vi "Update Digital Audio Generation (Freq and Amp)(N Chan).vi"(8 "error in (no error)":errorcluster, 9 "gain":dbl[](array[numeric]), 10 "frequency":dbl[](array[numeric]), 11 "PCM tasks":T1) -> (0 "error out":errorcluster, 3 "PCM tasks":T1)   [LabVIEW 2021]
uses:
  controls/digital audio protocol/PCM tasks.ctl
  <vilib>/PDM Acquisition Toolkit/host/Classes/Tasks/PCM Output/Controls/PCM Output Task DVR.ctl
  <vilib>/PDM Acquisition Toolkit/host/Classes/Tasks/PCM Output/PCM Output Task.lvclass
  C:/Program Files/National Instruments/LabVIEW 2021/vi.lib/PDM Acquisition Toolkit/host/Classes/Tasks/Parent/DecoderTask.lvclass
  <vilib>/PDM Acquisition Toolkit/host/Classes/Channels/PCM Output/PCM Output Channel.lvclass
  C:/Program Files/National Instruments/LabVIEW 2021/vi.lib/PDM Acquisition Toolkit/host/Classes/Channels/DecoderChannel.lvclass
  <vilib>/PDM Acquisition Toolkit/host/Classes/Channels/PCM Output/controls/PCM Output Channel - Signal Properties.ctl
  <vilib>/PDM Acquisition Toolkit/host/Classes/Channels/DecoderChannel.lvclass
  C:/Program Files/National Instruments/LabVIEW 2021/vi.lib/PDM Acquisition Toolkit/host/Classes/Channels/PCM Output/PCM Output Channel.lvclass
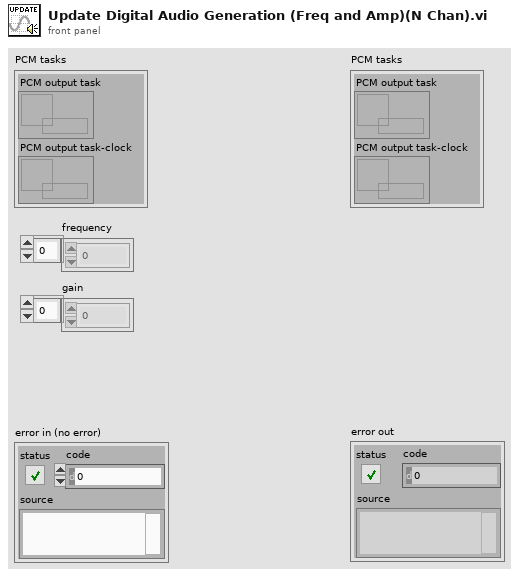
[diagram p1: front panel]
types:
  T1 = typedef "PCM tasks.ctl" = cluster{"PCM output task":T2, "PCM output task-clock":T2}
  T2 = typedef "PDM Acquisition Class Library.lvlib/PCM Output Task.lvclass/PCM Output Task DVR.ctl" = refnum<data-value>
  T3 = typedef "PDM Acquisition Class Library.lvlib/PCM Output Channel.lvclass/PCM Output Channel - Signal Properties.ctl" = cluster{"cyclic period":dbl, "cyclic phase offset":dbl, "gain":dbl}
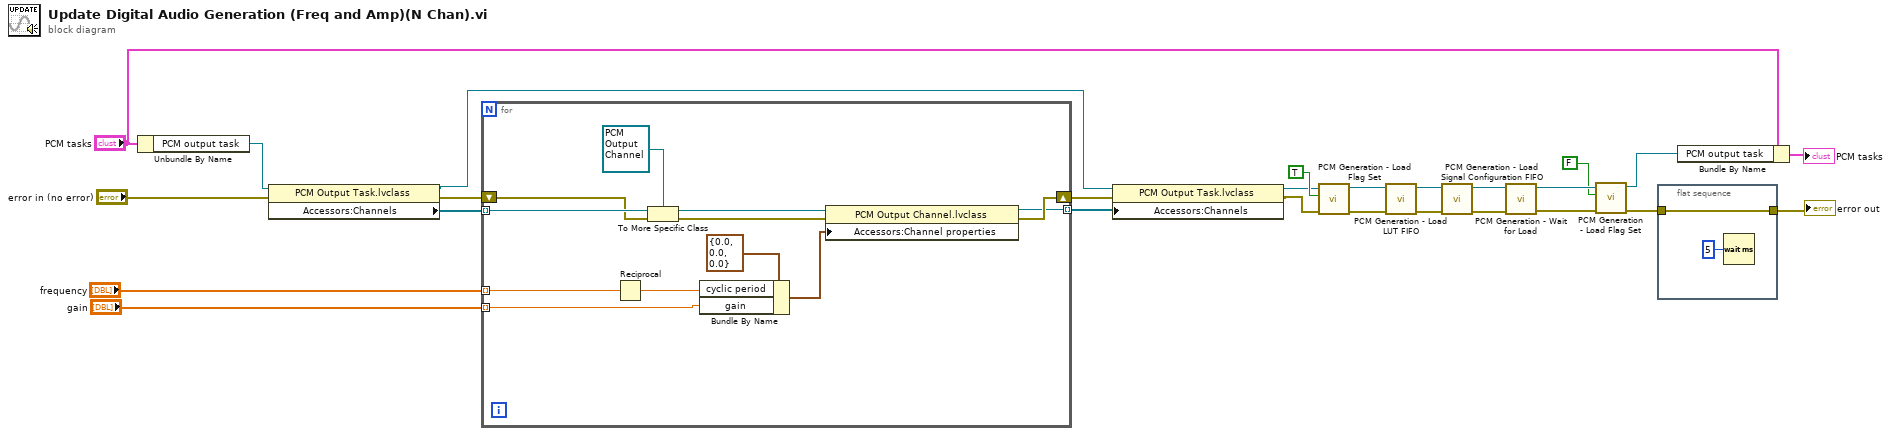
[diagram p0: block diagram]
diagram:
  n1 = Unbundle By Name("PCM tasks") -> ("PCM output task"=w8:T2)
  n2 = property class="PCM Output Task.lvclass"(reference=w8, error in="error in (no error)") -> (reference out=w13:T2, error out=w25:errorcluster, "Accessors:Channels"=w26:refnum<class "DecoderChannel.lvclass">[])
  n3 = for {
    tunnel: w26 -> [w37] mode=indexing
    shift-right: [w33] -> w15
    shift-left: w25 -> [w35]
    tunnel: [w32] -> w14 mode=indexing
    tunnel: "frequency" -> [w28] mode=indexing
    tunnel: "gain" -> [w27] mode=indexing
    n4 = Reciprocal(x=w28) -> (1/x=w31:dbl)
    n5 = To More Specific Class(target class=refnum<class "PCM Output Channel.lvclass"> refnum ("PDM Acquisition Class Library.lvlib:PCM Output Channel.lvclass"), reference=w37, error in=w35) -> (specific class reference=w34:refnum<class "PCM Output Channel.lvclass">, error out=w38:errorcluster)
    n6 = Bundle By Name(cluster=T3 {"cyclic period"=0.0, "cyclic phase offset"=0.0, "gain"=0.0} ("Channel properties"), "cyclic period"=w31, "gain"=w27) -> (w29:T3)
    n7 = property class="PCM Output Channel.lvclass"(reference=w34, error in=w38, "Accessors:Channel properties"=w29) -> (reference out=w32:refnum<class "PCM Output Channel.lvclass">, error out=w33:errorcluster)
  }
  n8 = property class="PCM Output Task.lvclass"(reference=w13, error in=w15, "Accessors:Channels"=w14) -> (reference out=w12:T2, error out=w11:errorcluster)
  n9 = call <vilib>:"PCM Generation - Load Flag Set.vi"("error in"=w11, "Load"=TRUE, "PCM Output Task In"=w12) -> ("error out"=w19:errorcluster, "PCM Output Task Out"=w18:T2)  [unwired: 7 in]
  n10 = call <vilib>:"PCM Generation - Load LUT FIFO.vi"("error in"=w19, "PCM Output Task In"=w18) -> ("error out"=w16:errorcluster, "PCM Output Task Out"=w17:T2)  [unwired: 8 in]
  n11 = call <vilib>:"PCM Generation - Load Signal Configuration FIFO.vi"("error in"=w16, "PCM Output Task In"=w17) -> ("error out"=w10:errorcluster, "PCM Output Task Out"=w20:T2)  [unwired: 8 in]
  n12 = call <vilib>:"PCM Generation - Wait for Load.vi"("error in"=w10, "PCM Output Task In"=w20) -> ("error out"=w22:errorcluster, "PCM Output Task Out"=w23:T2)  [unwired: 7 in, 1 out]
  n13 = call <vilib>:"PCM Generation - Load Flag Set.vi"("error in"=w22, "Load"=FALSE, "PCM Output Task In"=w23) -> ("error out"=w4:errorcluster, "PCM Output Task Out"=w5:T2)  [unwired: 7 in]
  n14 = flat-sequence {
    tunnel: w4 -> [w40]
    tunnel: [w40] -> w3
    frame #0 {
      n15 = Wait (ms)(milliseconds to wait=u32 5) -> ()  [unwired: 1 out]
    }
  }
  n16 = Bundle By Name(cluster="PCM tasks", "PCM output task"=w5) -> (→"PCM tasks":T1)
  "error out" <- w3
